vi "Read Digital Config.vi"(8 "error in (no error)":errorcluster) -> (0 "error out":errorcluster, 3 "Señal Digital":T1={"Puertos/Pines"="", "Puerto"="DAQSim1", "Pines"=[], "Tiempo de AQ"=0.0, "Tiempo entre AQ"=0.0})   [LabVIEW 2020, in "Settings.lvlib"]
uses:
  Settings.lvlib
  Aqcisition/Digital Signal Config.ctl
  <vilib>/drjdpowell/SQLite Library/SQL Connection/Open (path).vi
  <vilib>/drjdpowell/SQLite Library/SQL Connection/Open (string).vi
  <vilib>/AdvancedString/Path To Command Line String.vi
  <vilib>/drjdpowell/SQLite Library/SQL Connection/Execute SQL (1D String).vi
  <vilib>/drjdpowell/SQLite Library/SQL Connection/Connection.lvclass
  <vilib>/drjdpowell/SQLite Library/SQLite.lvlib
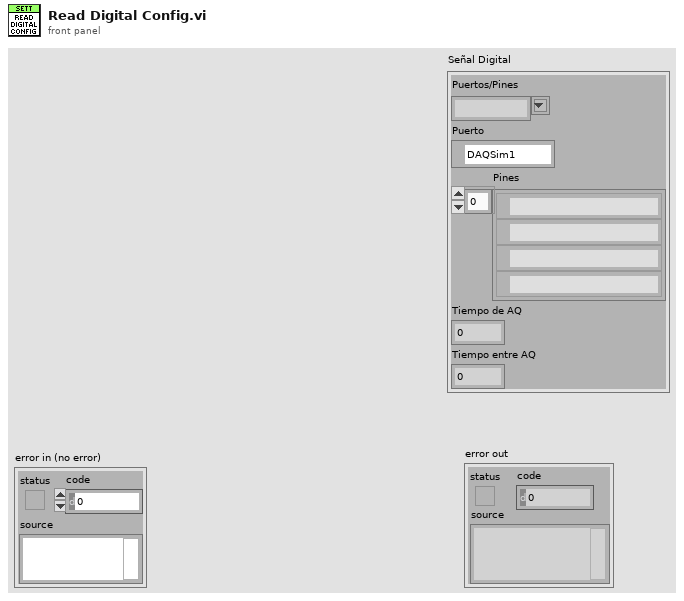
[diagram p1: front panel]
types:
  T1 = typedef "Digital Signal Config.ctl" = cluster{"Puertos/Pines":string, "Puerto":tag, "Pines":tag[], "Tiempo de AQ":dbl, "Tiempo entre AQ":dbl}
  T2 = cluster{"Text":string, "Text":string, "Text":string, "Text":string}
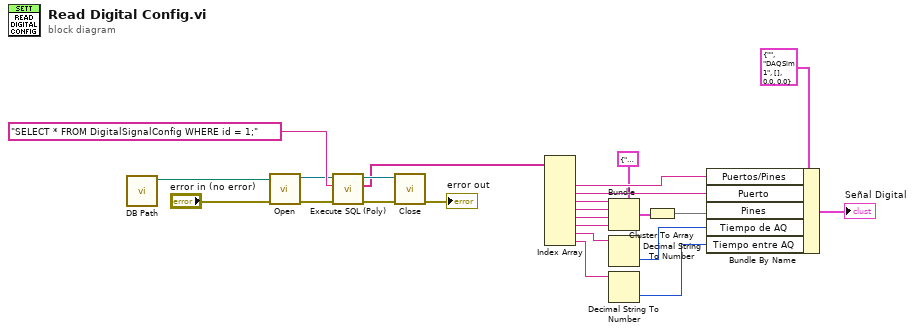
[diagram p0: block diagram]
diagram:
  n1 = call "DB Path.vi"() -> ("appended path"=w16:path)  [unwired: 11 in]
  n2 = call-poly <vilib>:"Open.vi"("error in (no error)"="error in (no error)", "db file"=w16) -> ("error out"=w24:errorcluster, "SQLite Connection"=w19:refnum<class "Connection.lvclass">)  [unwired: 8 in]
  n3 = call-poly <vilib>:"Execute SQL (Poly).vi"("error in (no error)"=w24, "SQL"="SELECT * FROM DigitalSignalConfig WHERE id = 1;", "SQLite Connection in"=w19) -> ("error out"=w23:errorcluster, "Result Set"=w17:string[], "SQLite Connection"=w18:refnum<class "Connection.lvclass">)  [unwired: 5 in, 1 out]
  n4 = call-dynamic "Close.vi"("error in (no error)"=w23, "SQLite Connection in"=w18) -> ("error out"=→"error out":errorcluster)  [unwired: 9 in]
  n5 = Index Array(array=w17) -> (element #2=w12:string, element #3=w13:string, element #4=w9:string, element #5=w8:string, element #6=w7:string, element #7=w6:string, element #8=w4:string, element #9=w3:string)  [unwired: 9 in, 1 out]
  n6 = Bundle(cluster=T2 {"Text"="", "Text"="", "Text"="", "Text"=""}, "Text"=w9, "Text"=w8, "Text"=w7, "Text"=w6) -> (w10:T2)
  n7 = Decimal String To Number(string=w4) -> (number=w2:i32)  [unwired: 2 in, 1 out]
  n8 = Decimal String To Number(string=w3) -> (number=w1:i32)  [unwired: 2 in, 1 out]
  n9 = Cluster To Array(cluster=w10) -> (array=w5:string[])
  n10 = Bundle By Name(cluster=T1 {"Puertos/Pines"="", "Puerto"="DAQSim1", "Pines"=[], "Tiempo de AQ"=0.0, "Tiempo entre AQ"=0.0} ("Señal Digital"), "Puertos/Pines"=w12, "Puerto"=w13, "Pines"=w5, "Tiempo de AQ"=w2, "Tiempo entre AQ"=w1) -> (→"Señal Digital":T1)
